vi "Flush Action Queue.vi"(0 "action queue in":refnum<queue>, 11 "error in":errorcluster) -> (4 "action queue out":refnum<queue>, 8 "remaining actions":T1[](array[typedef]), 15 "error out":errorcluster)   [LabVIEW 2023, in "TLB` InstStu GPlugin Template.lvlib" / "Actions.lvlib"]
doc: "create queue resource for MAIN communication.\n\n<B>Input Parameters</B>\n\n<B>error in</B> describes error conditions that occur before this node runs. This input provides standard error in functionality.\n\n<B>Output Parameters</B>\n\n<B>MAIN-Trigger Queue out</B> trigger queue reference.\n\n<B>error out</B> contains error information. This output provides standard error out functionality."
uses:
  Actions.lvlib
  System Action Element.ctl
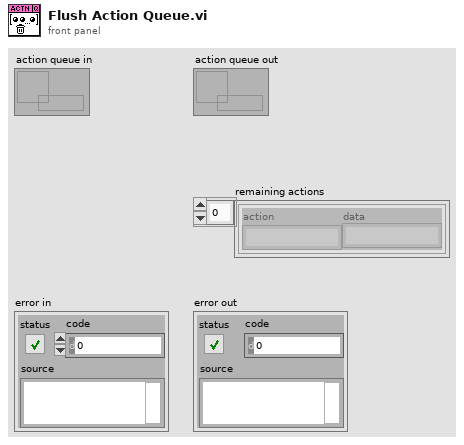
[diagram p1: front panel]
types:
  T1 = typedef "TLB` InstStu GPlugin Template.lvlib/Actions.lvlib/System Action Element.ctl" = cluster{"action":string, "data":string}
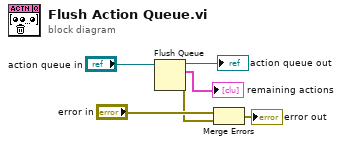
[diagram p0: block diagram]
diagram:
  n1 = Flush Queue(queue="action queue in") -> (queue out=→"action queue out":refnum<queue>, remaining elements=→"remaining actions":T1[], error out=w4:errorcluster)  [unwired: 1 in]
  n2 = Merge Errors("error in", w4) -> (→"error out":errorcluster)
